vi "6-3.vi"() -> ()   [LabVIEW 2017]
uses:
  <vilib>/measure/NI_MABase.lvlib
panel:
  out "signal out":waveform(dbl) caption="信号输出"
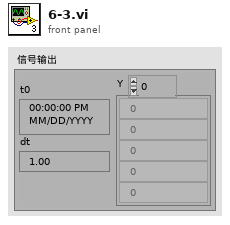
[diagram p1: front panel]
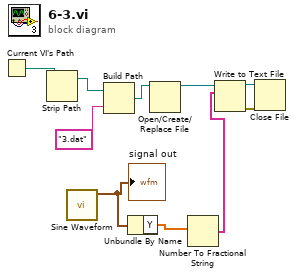
[diagram p0: block diagram]
diagram:
  n1 = Current VI's Path() -> (path=w2:path)
  n2 = Strip Path(path=w2) -> (stripped path=w1:path)  [unwired: 1 out]
  n3 = call <vilib>:"Sine Waveform.vi"() -> ("signal out"=w5:waveform(dbl))  [unwired: 10 in, 1 out]
  "signal out" <- w5
  n4 = Build Path(base path=w1, name or relative path="3.dat" ("名称或相对路径")) -> (appended path=w9:path)
  n5 = Unbundle By Name(w5) -> ("Y"=w4:dbl[])
  n6 = Open/Create/Replace File(file path (use dialog)=w9) -> (refnum out=w6:refnum<file>)  [unwired: 5 in, 2 out]
  n7 = Number To Fractional String(number=w4) -> (F-format string=w3:string[])  [unwired: 3 in]
  n8 = Write to Text File(file (use dialog)=w6, text=w3) -> (refnum out=w7:refnum<file>, error out=w8:errorcluster)  [unwired: 2 in, 1 out]
  n9 = Close File(refnum=w7, error in=w8) -> ()  [unwired: 2 out]
